vi "Intake Globals.vi"() -> ()   [LabVIEW 2016]
uses:
  Intake Notifier.ctl
  Intake Control Type.ctl
panel:
  in  "Intake Motor":string="Intake Motor"
  in  "Intake DVR":refnum<data-value>
  in  "Intake Notifier":refnum<notifier>
  # "These refnums are for the writing and creation\nof the intake subsystem's data."
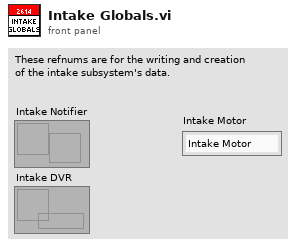
[diagram p1: front panel]
diagram:
